vi "Banana_Equal Value Comparison.vi"(6 "verbose? (F)":bool, 8 "error in (no error)":errorcluster, 9 "Y":variant, 10 "X":variant) -> (0 "error out":errorcluster, 2 "Equal Values?":bool, 3 "Verbose output":string)   [LabVIEW 2021, in "Bananas.lvlib"]
uses:
  Bananas.lvlib
  <vilib>/LabVIEW Open Source Project/Data Manipulation/TypeDescriptor/TypeDescriptor_GetType.vi
  <vilib>/LabVIEW Open Source Project/Data Manipulation/TypeDescriptor/TypeDescriptor_GetName.vi
  <vilib>/LabVIEW Open Source Project/Data Manipulation/TypeDescriptor/TypeDescriptor_GetPString.vi
  <vilib>/LabVIEW Open Source Project/Data Manipulation/Conversions/Flattened nD-Array to Flattened 1D-Array.vi
  <vilib>/Utility/Data Type/NI_Data Type.lvlib
  <vilib>/LabVIEW Open Source Project/Data Manipulation/Variant/OpenVariant.lvlib
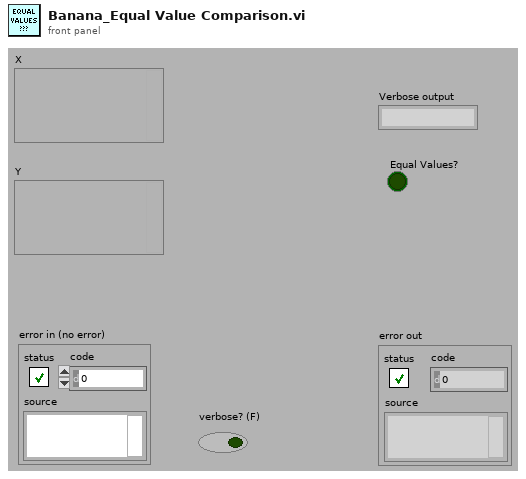
[diagram p1: front panel]
types:
  T1 = typedef "NI_Data Type.lvlib/Data Type.ctl" = enum8{"Invalid Type", "Void", "I8", "I16", "I32", "I64", "U8", "U16", "U32", "U64", "Single Float", "Double Float", "Extended Float", "Single Complex", "Double Complex", "Extended Complex", "Enum U8", "Enum U16", "Enum U32", "Enum U64", "Single Float With Unit", "Double Float With Unit", "Extended Float With Unit", "Single Complex with Unit", "Double Complex with Unit", "Extended Complex with Unit", "Boolean", "String", "Path", "Picture", "Tag", "Array", "Cluster", "Variant", "LV Variant", "Waveform", "Timestamp", "Digital Waveform", "Digital Data", "ExpressData", "Refnum", "External Data", "VI", "Poly VI", "LabVIEW Class Instance", "Fixed Point", "Set Collection", "Map Collection"}
  T2 = typedef "NI_Data Type.lvlib/Unit Info.ctl" = cluster{"Unit Type":T3, "Exponent":i16}
  T3 = typedef "NI_Data Type.lvlib/Unit Type.ctl" = enum16{"Radians", "Steradians", "Seconds", "Meters", "Kilograms", "Amperes", "Kelvins", "Moles", "Candelas", "InvalidUnit"}
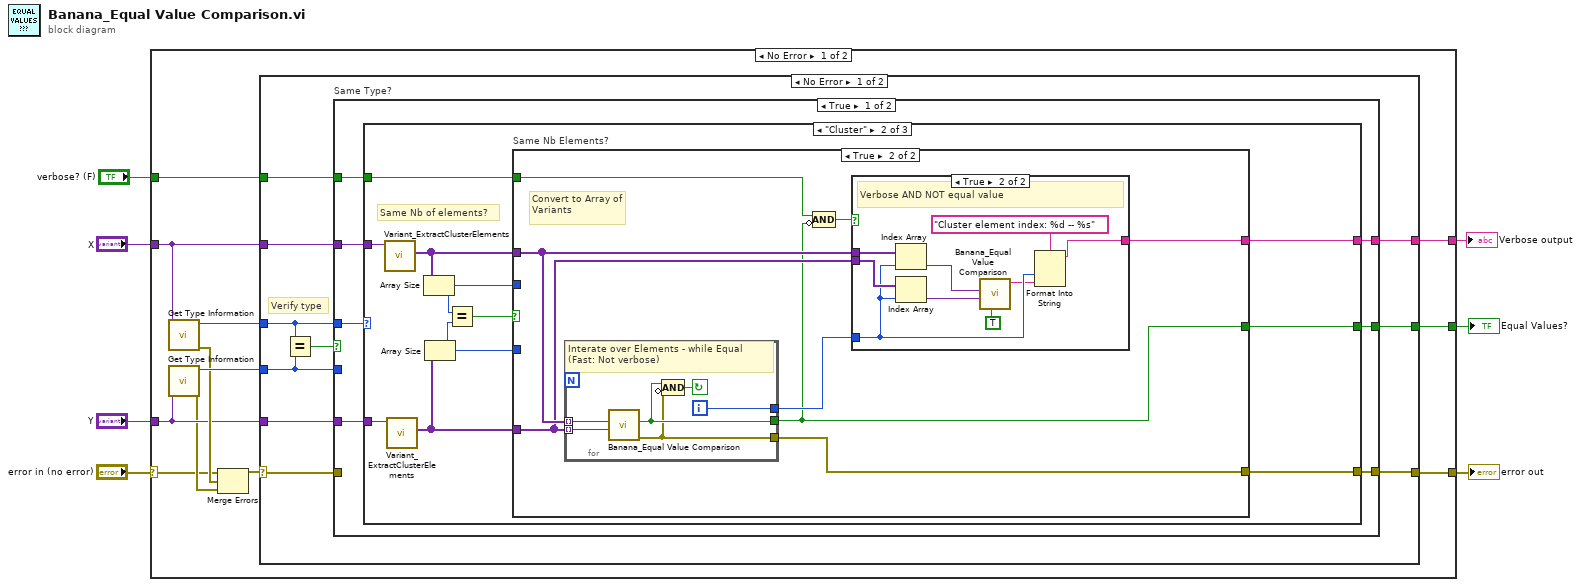
[diagram p0: block diagram]
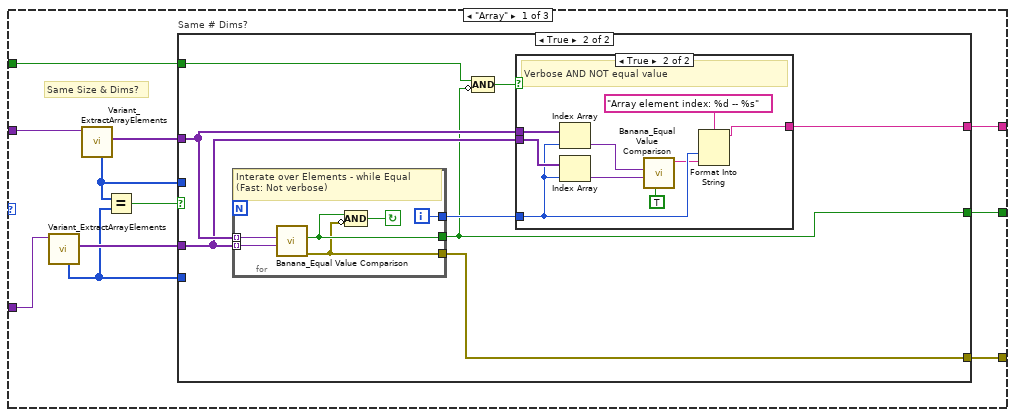
[diagram p2: hidden frame]
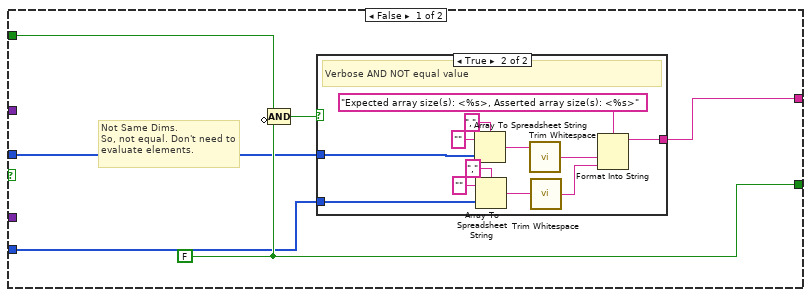
[diagram p3: hidden frame]
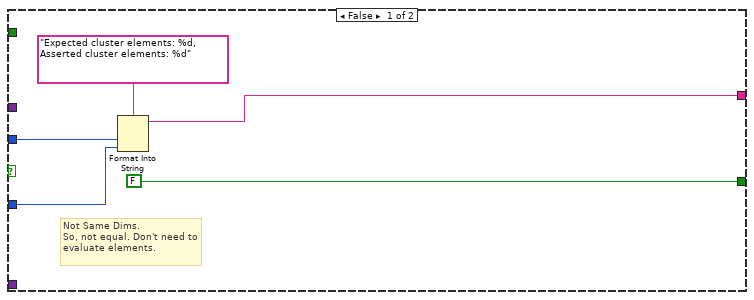
[diagram p6: hidden frame]
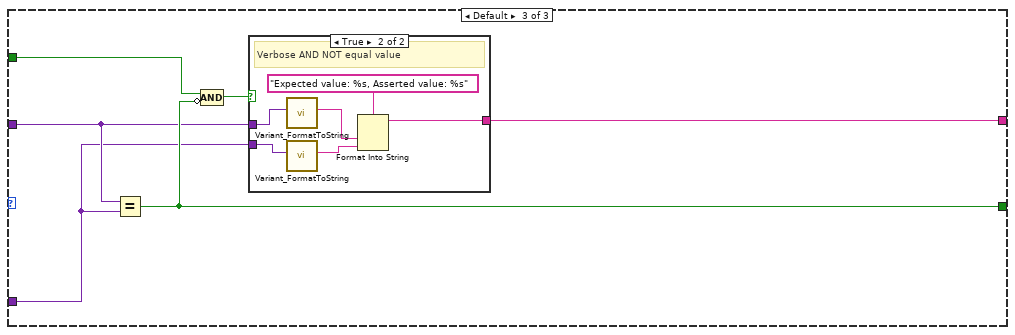
[diagram p8: hidden frame]
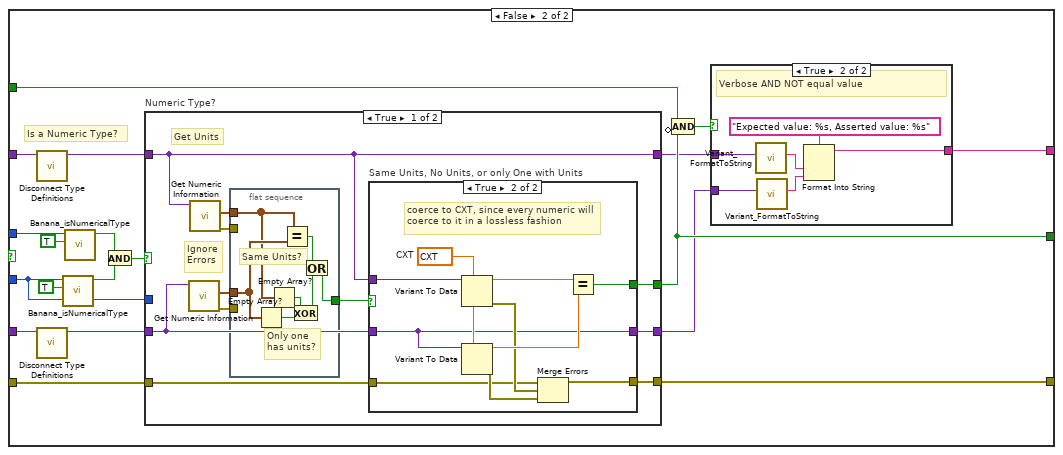
[diagram p10: hidden frame]
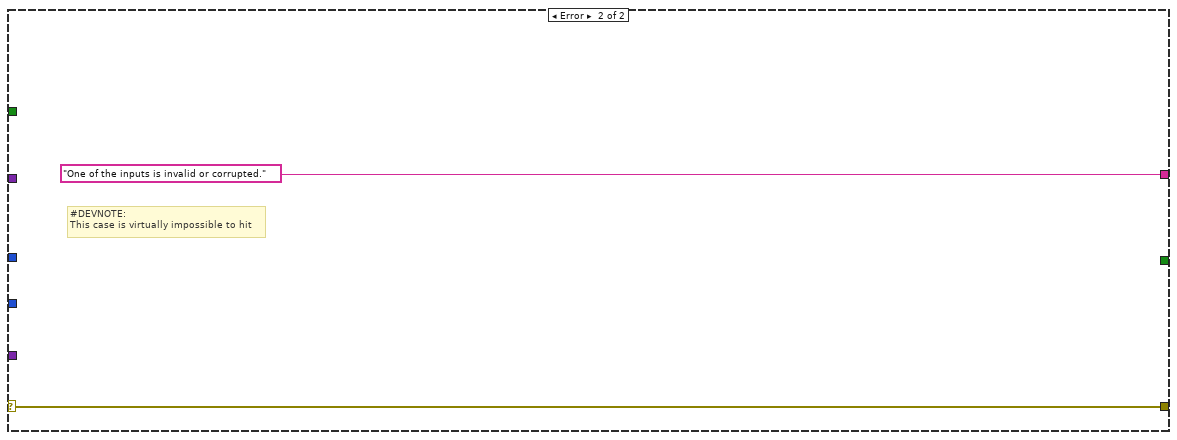
[diagram p14: hidden frame]
diagram:
  n1 = case shown="No Error" "error in (no error)" {
    selector: "error in (no error)" -> [w8 w198]
    tunnel: [w19 _] -> w7
    tunnel: [w18 w198] -> w6
    tunnel: "Y" -> [w11 _]
    tunnel: "X" -> [w13 _]
    tunnel: "verbose? (F)" -> [w17 _]
    tunnel: [w16 _] -> w2
    frame No Error {
      n2 = call <vilib>:"Get Type Information.vi"("variant"=w13) -> ("error out"=w12:errorcluster, "type"=w14:T1)  [unwired: 6 in, 3 out]
      n3 = call <vilib>:"Get Type Information.vi"("variant"=w11) -> ("error out"=w9:errorcluster, "type"=w15:T1)  [unwired: 6 in, 3 out]
      n4 = Merge Errors(w8, w12, w9) -> (w10:errorcluster)
      n5 = case shown="No Error" w10 {
        selector: w10 -> [w20 w197]
        tunnel: [w29 _] -> w19
        tunnel: [w28 w197] -> w18
        tunnel: w17 -> [w27 _]
        tunnel: [w26 "One of the inputs is invalid or corrupted." ("format string")] -> w16
        tunnel: w15 -> [w25 _]
        tunnel: w14 -> [w24 _]
        tunnel: w13 -> [w23 _]
        tunnel: w11 -> [w21 _]
        frame No Error {
          # "Verify type"
          n6 = Equal?(x=w24, y=w25) -> (x = y?=w22:bool)
          n7 = case "Same Type?" shown="True" w22 {
            tunnel: w23 -> [w34 w151]
            tunnel: w21 -> [w33 w149]
            tunnel: [w36 w155] -> w29
            tunnel: w24 -> [w35 w143]
            tunnel: w25 -> [_ w147]
            tunnel: [w32 w158] -> w28
            tunnel: w27 -> [w31 w156]
            tunnel: [w30 w140] -> w26
            tunnel: w20 -> [_ w141]
            frame True {
              n8 = case shown="\"Cluster\"" w35 {
                tunnel: [w46 w99 w133] -> w36
                tunnel: w34 -> [w40 w92 w129]
                tunnel: w33 -> [w39 w91 w128]
                tunnel: [w47 w98 _] -> w32
                tunnel: w31 -> [w45 w96 w132]
                tunnel: [w44 w93 w130] -> w30
                frame "Array" {
                  # "Same Size & Dims?"
                  n9 = call <vilib>:"Variant_ExtractArrayElements.vi"("Array"=w39) -> ("Elements"=w38:variant[], "Dimensions"=w37:u32[])  [unwired: 7 in, 2 out]
                  n10 = call <vilib>:"Variant_ExtractArrayElements.vi"("Array"=w40) -> ("Elements"=w43:variant[], "Dimensions"=w42:u32[])  [unwired: 7 in, 2 out]
                  n11 = Equal?(x=w42, y=w37) -> (x = y?=w41:bool)
                  n12 = case "Same # Dims?" shown="True" w41 {
                    tunnel: [w51 w66] -> w46
                    tunnel: [_ w68] -> w47
                    tunnel: w45 -> [w52 w72]
                    tunnel: [w50 w71] -> w44
                    tunnel: w42 -> [w49 _]
                    tunnel: w37 -> [w48 _]
                    tunnel: w43 -> [_ w70]
                    tunnel: w38 -> [_ w69]
                    frame False {
                      w51 = FALSE ("Equal Values?")
                      # "Not Same Dims.\nSo, not equal. Don't need to evaluate elements."
                      n13 = Compound Arithmetic op=AND(w52, invert w51) -> (w53:bool)
                      n14 = case shown="True" w53 {
                        tunnel: [_ w65] -> w50
                        tunnel: w49 -> [_ w55]
                        tunnel: w48 -> [_ w54]
                        frame False {
                        }
                        frame True {
                          # "Verbose AND NOT equal value"
                          n15 = Array To Spreadsheet String(delimiter (Tab)=",", array=w55, 3:"" ("format string")) -> (spreadsheet string=w61:string)
                          n16 = Array To Spreadsheet String(delimiter (Tab)=",", array=w54, 3:"" ("format string")) -> (spreadsheet string=w59:string)
                          n17 = call <vilib>:"Trim Whitespace.vi"("string"=w61) -> ("trimmed string"=w60:string)  [unwired: 1 in]
                          n18 = call <vilib>:"Trim Whitespace.vi"("string"=w59) -> ("trimmed string"=w56:string)  [unwired: 1 in]
                          n19 = Format Into String(format string="Expected array size(s): <%s>, Asserted array size(s): <%s>", w60, w56) -> (resulting string=w65:string)  [unwired: 2 in, 1 out]
                        }
                      }
                    }
                    frame True {
                      n20 = for {
                        tunnel: w70 -> [w88] mode=indexing
                        tunnel: w69 -> [w87] mode=indexing
                        tunnel: [w86] -> w66
                        tunnel: [w84] -> w68
                        tunnel: [w83] -> w67
                        i -> [w83]
                        stop <- w85 continue-if-true
                        # "Interate over Elements - while Equal\n(Fast: Not verbose)"
                        n21 = call "Banana_Equal Value Comparison.vi"("Y"=w87, "X"=w88) -> ("error out"=w84:errorcluster, "Equal Values?"=w86:bool)  [unwired: 7 in, 1 out]
                        n22 = Compound Arithmetic op=AND(w86, invert w84) -> (w85:bool)
                      }
                      n23 = Compound Arithmetic op=AND(w72, invert w66) -> (w73:bool)
                      n24 = case shown="True" w73 {
                        tunnel: [_ w81] -> w71
                        tunnel: w70 -> [_ w80]
                        tunnel: w69 -> [_ w79]
                        tunnel: w67 -> [_ w75]
                        frame False {
                        }
                        frame True {
                          # "Verbose AND NOT equal value"
                          n25 = Index Array(array=w80, index=w75) -> (element=w76:variant)
                          n26 = Index Array(array=w79, index=w75) -> (element=w77:variant)
                          n27 = call "Banana_Equal Value Comparison.vi"("verbose? (F)"=TRUE, "Y"=w77, "X"=w76) -> ("Verbose output"=w74:string)  [unwired: 6 in, 2 out]
                          n28 = Format Into String(format string="Array element index: %d -- %s", w75, w74) -> (resulting string=w81:string)  [unwired: 2 in, 1 out]
                        }
                      }
                    }
                  }
                }
                frame "Cluster" {
                  # "Same Nb of elements?"
                  n29 = call <vilib>:"Variant_ExtractClusterElements.vi"("Cluster"=w92) -> ("Elements"=w90:variant[])  [unwired: 8 in, 2 out]
                  n30 = call <vilib>:"Variant_ExtractClusterElements.vi"("Cluster"=w91) -> ("Elements"=w89:variant[])  [unwired: 8 in, 2 out]
                  n31 = Array Size(array=w90) -> (size(s)=w95:i32)
                  n32 = Array Size(array=w89) -> (size(s)=w94:i32)
                  n33 = Equal?(x=w95, y=w94) -> (x = y?=w97:bool)
                  n34 = case "Same Nb Elements?" shown="True" w97 {
                    tunnel: [FALSE ("Equal Values?") w106] -> w99
                    tunnel: [_ w105] -> w98
                    tunnel: w96 -> [_ w112]
                    tunnel: w95 -> [w103 _]
                    tunnel: w94 -> [w102 _]
                    tunnel: [w100 w107] -> w93
                    tunnel: w90 -> [_ w110]
                    tunnel: w89 -> [_ w109]
                    frame False {
                      # "Not Same Dims.\nSo, not equal. Don't need to evaluate elements."
                      n35 = Format Into String(format string="Expected cluster elements: %d, Asserted cluster elements: %d", w103, w102) -> (resulting string=w100:string)  [unwired: 2 in, 1 out]
                    }
                    frame True {
                      # "Convert to Array of Variants"
                      n36 = for {
                        tunnel: w110 -> [w127] mode=indexing
                        tunnel: w109 -> [w126] mode=indexing
                        tunnel: [w125] -> w106
                        tunnel: [w123] -> w105
                        tunnel: [w122] -> w108
                        i -> [w122]
                        stop <- w124 continue-if-true
                        # "Interate over Elements - while Equal\n(Fast: Not verbose)"
                        n37 = call "Banana_Equal Value Comparison.vi"("Y"=w126, "X"=w127) -> ("error out"=w123:errorcluster, "Equal Values?"=w125:bool)  [unwired: 7 in, 1 out]
                        n38 = Compound Arithmetic op=AND(w125, invert w123) -> (w124:bool)
                      }
                      n39 = Compound Arithmetic op=AND(w112, invert w106) -> (w111:bool)
                      n40 = case shown="True" w111 {
                        tunnel: [_ w120] -> w107
                        tunnel: w110 -> [_ w119]
                        tunnel: w109 -> [_ w118]
                        tunnel: w108 -> [_ w114]
                        frame False {
                        }
                        frame True {
                          # "Verbose AND NOT equal value"
                          n41 = Index Array(array=w119, index=w114) -> (element=w115:variant)
                          n42 = Index Array(array=w118, index=w114) -> (element=w116:variant)
                          n43 = call "Banana_Equal Value Comparison.vi"("verbose? (F)"=TRUE, "Y"=w116, "X"=w115) -> ("Verbose output"=w113:string)  [unwired: 6 in, 2 out]
                          n44 = Format Into String(format string="Cluster element index: %d -- %s", w114, w113) -> (resulting string=w120:string)  [unwired: 2 in, 1 out]
                        }
                      }
                    }
                  }
                }
                frame Default {
                  n45 = Equal?(x=w129, y=w128) -> (x = y?=w133:bool)
                  n46 = Compound Arithmetic op=AND(w132, invert w133) -> (w131:bool)
                  n47 = case shown="True" w131 {
                    tunnel: [_ w139] -> w130
                    tunnel: w129 -> [_ w137]
                    tunnel: w128 -> [_ w134]
                    frame False {
                    }
                    frame True {
                      # "Verbose AND NOT equal value"
                      n48 = call <vilib>:"Variant_FormatToString.vi"("Variant"=w137) -> ("Value"=w136:string)  [unwired: 10 in]
                      n49 = call <vilib>:"Variant_FormatToString.vi"("Variant"=w134) -> ("Value"=w135:string)  [unwired: 10 in]
                      n50 = Format Into String(format string="Expected value: %s, Asserted value: %s", w136, w135) -> (resulting string=w139:string)  [unwired: 2 in, 1 out]
                    }
                  }
                }
              }
            }
            frame False {
              # "Is a Numeric Type?"
              n51 = call <vilib>:"Disconnect Type Definitions.vi"("variant in"=w151) -> ("variant out"=w150:variant)  [unwired: 9 in, 1 out]
              n52 = call <vilib>:"Disconnect Type Definitions.vi"("variant in"=w149) -> ("variant out"=w148:variant)  [unwired: 9 in, 1 out]
              n53 = call "Banana_isNumericalType.vi"("Allow Complex?"=TRUE, "Type Enum"=w147) -> ("is Numeric"=w145:bool)  [unwired: 9 in]
              n54 = call "Banana_isNumericalType.vi"("Allow Complex?"=TRUE, "Type Enum"=w143) -> ("is Numeric"=w142:bool)  [unwired: 9 in]
              n55 = And(x=w142, y=w145) -> (x .and. y?=w157:bool)
              n56 = case "Numeric Type?" shown="True" w157 {
                tunnel: w150 -> [w172 w195]
                tunnel: w148 -> [w166 w194]
                tunnel: w147 -> [_ _]
                tunnel: [w175 _] -> w155
                tunnel: [w174 _] -> w158
                tunnel: [w172 w195] -> w153
                tunnel: [w165 w194] -> w152
                tunnel: w141 -> [w167 _]
                frame True {
                  # "Get Units"
                  # "Ignore\nErrors"
                  n57 = call <vilib>:"Get Numeric Information.vi"("variant"=w166) -> ("error out"=w168:errorcluster, "units"=w171:T2[])  [unwired: 7 in, 2 out]
                  n58 = call <vilib>:"Get Numeric Information.vi"("variant"=w172) -> ("error out"=w169:errorcluster, "units"=w170:T2[])  [unwired: 7 in, 2 out]
                  n59 = flat-sequence {
                    tunnel: w170 -> [w192]
                    tunnel: w171 -> [w193]
                    tunnel: [w187] -> w173
                    tunnel: w169 -> [_]
                    tunnel: w168 -> [_]
                    frame #0 {
                      # "Same Units?"
                      # "Only one\nhas units?"
                      n60 = Empty Array?(array=w193) -> (empty?=w191:bool)
                      n61 = Empty Array?(array=w192) -> (empty?=w190:bool)
                      n62 = Equal?(x=w192, y=w193) -> (x = y?=w188:bool)
                      n63 = Exclusive Or(1:w191, 2:w190) -> (0:w189:bool)
                      n64 = Or(x=w188, y=w189) -> (x .or. y?=w187:bool)
                    }
                  }
                  n65 = case "Same Units, No Units, or only One with Units" shown="True" w173 {
                    tunnel: [_ w186] -> w175
                    tunnel: [_ w179] -> w174
                    tunnel: w172 -> [_ w182]
                    tunnel: w166 -> [w176 w177]
                    tunnel: w167 -> [_ w178]
                    tunnel: [w176 w177] -> w165
                    frame False {
                      # "Different Units\nCannot have equal value"
                    }
                    frame True {
                      w183 = cxt 0.0+0.0i  # CXT
                      # "coerce to CXT, since every numeric will coerce to it in a lossless fashion"
                      n66 = Variant To Data(type=w183, Variant=w182) -> (data=w185:cxt, error out=w181:errorcluster)  [unwired: 1 in]
                      n67 = Variant To Data(type=w183, Variant=w177) -> (data=w184:cxt, error out=w180:errorcluster)  [unwired: 1 in]
                      n68 = Merge Errors(w178, w181, w180) -> (w179:errorcluster)
                      n69 = Equal?(x=w185, y=w184) -> (x = y?=w186:bool)
                    }
                  }
                }
                frame False {
                  # "All non-integer representations must be of same type to potentially assert True,"
                }
              }
              n70 = Compound Arithmetic op=AND(w156, invert w155) -> (w154:bool)
              n71 = case shown="True" w154 {
                tunnel: [_ w164] -> w140
                tunnel: w153 -> [_ w162]
                tunnel: w152 -> [_ w160]
                frame False {
                }
                frame True {
                  # "Verbose AND NOT equal value"
                  n72 = call <vilib>:"Variant_FormatToString.vi"("Variant"=w162) -> ("Value"=w161:string)  [unwired: 10 in]
                  n73 = call <vilib>:"Variant_FormatToString.vi"("Variant"=w160) -> ("Value"=w159:string)  [unwired: 10 in]
                  n74 = Format Into String(format string="Expected value: %s, Asserted value: %s", w161, w159) -> (resulting string=w164:string)  [unwired: 2 in, 1 out]
                }
              }
            }
          }
        }
        frame Error {
          # "#DEVNOTE: \nThis case is virtually impossible to hit"
        }
      }
    }
    frame Error {
    }
  }
  "Equal Values?" <- w7
  "error out" <- w6
  "Verbose output" <- w2
